vi "read_sample_results_files.vi"(8 "Error In":errorcluster, 10 "Sample":string, 11 "File Path":path) -> (0 "Error Out":errorcluster, 3 "Sample Results":T1)   [LabVIEW 2019]
uses:
  sample_results_cluster_typedef.ctl
  parameters_cluster_typedef.ctl
  writeable_section_parameters_cluster_typedef.ctl
  grain_results_cluster_typedef.ctl
panel:
  out "Exists?":bool
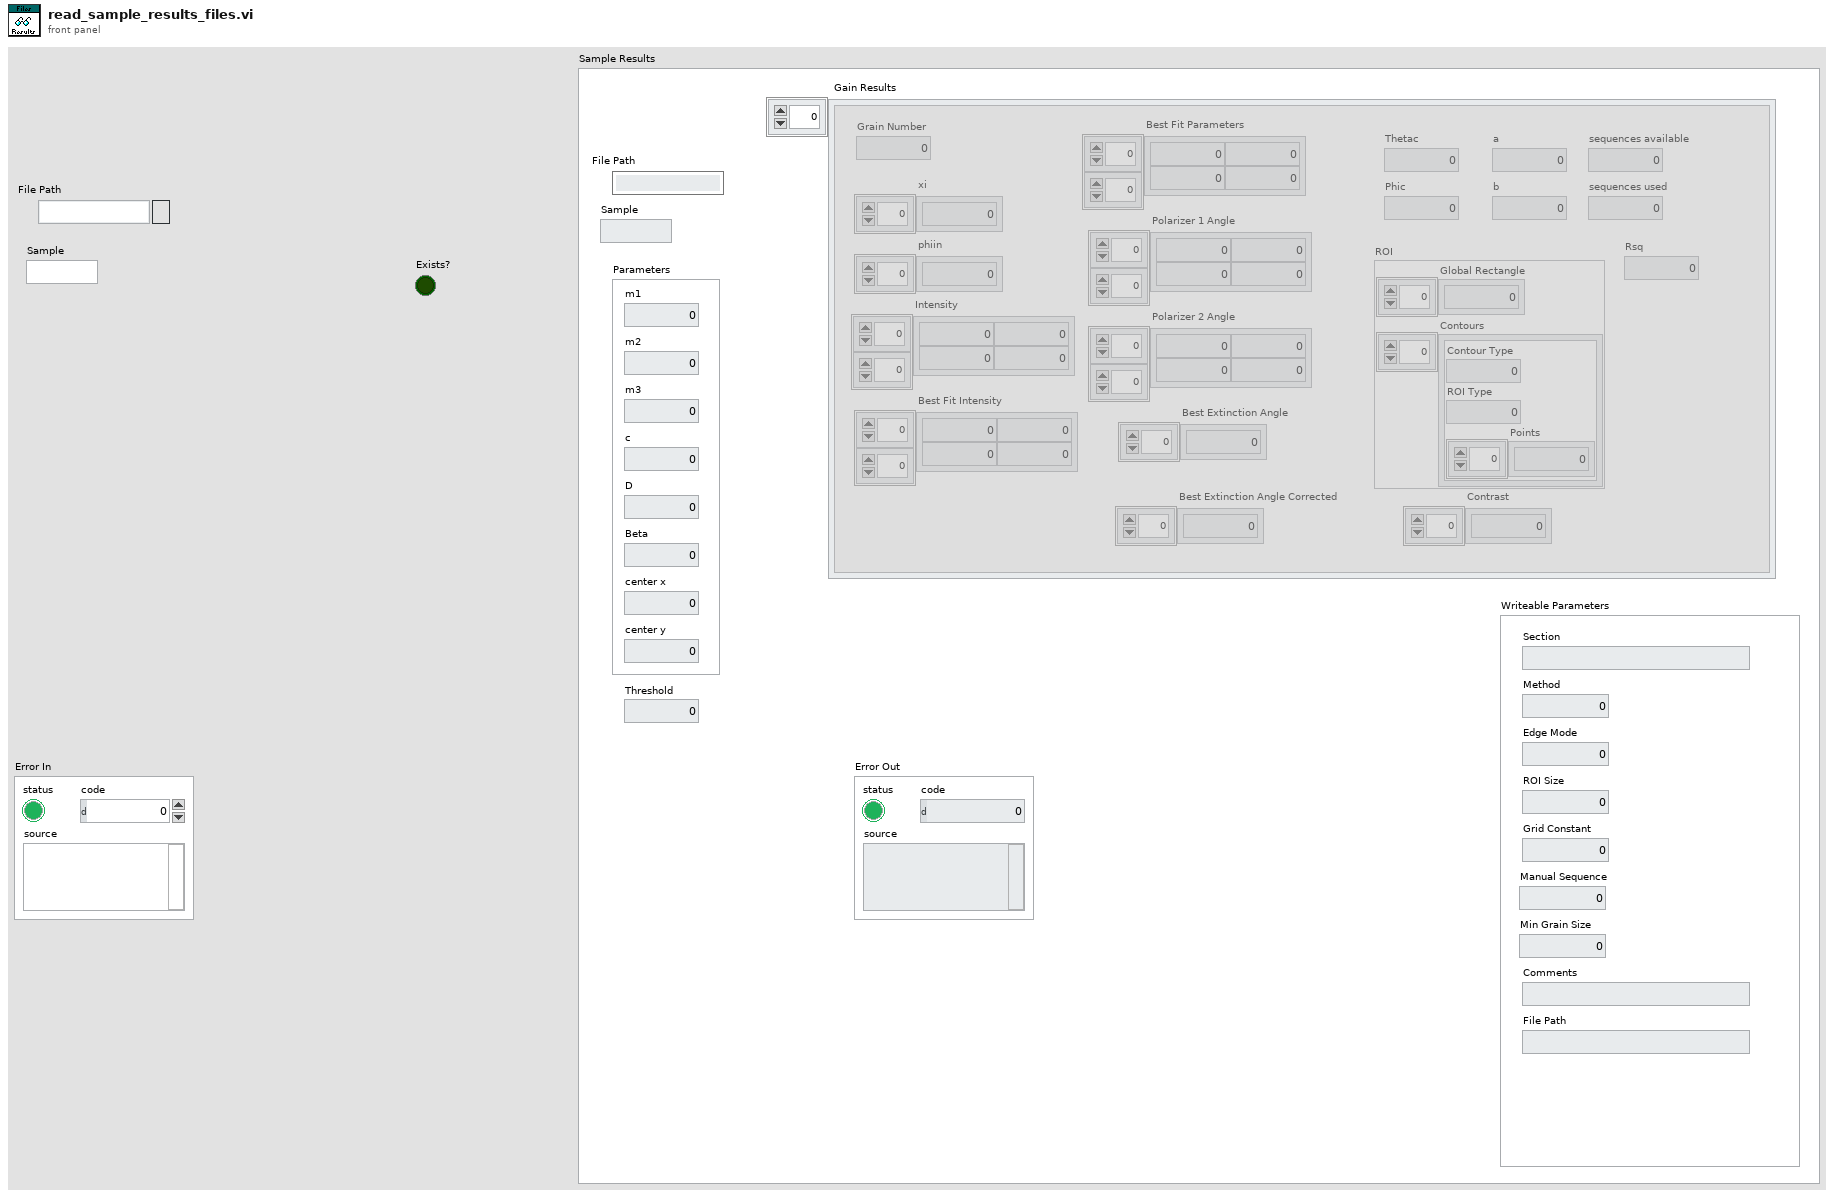
[diagram p1: front panel]
types:
  T1 = typedef "sample_results_cluster_typedef.ctl" = cluster{"File Path":string, "Sample":string, "Threshold":dbl, "Parameters":T2, "Writeable Parameters":T3, "Gain Results":T4[]}
  T2 = typedef "parameters_cluster_typedef.ctl" = cluster{"m1":dbl, "m2":dbl, "m3":dbl, "c":dbl, "D":dbl, "Beta":dbl, "center x":dbl, "center y":dbl}
  T3 = typedef "writeable_section_parameters_cluster_typedef.ctl" = cluster{"Section":string, "Method":i32, "Edge Mode":i32, "Grid Constant":i32, "Manual Sequence":i32, "ROI Size":i32, "Min Grain Size":dbl, "Comments":string, "File Path":string}
  T4 = typedef "grain_results_cluster_typedef.ctl" = cluster{"Grain Number":i32, "xi":dbl[], "phiin":dbl[], "Intensity":dbl[][], "Best Fit Intensity":dbl[][], "Best Fit Parameters":dbl[][], "Polarizer 1 Angle":dbl[][], "Polarizer 2 Angle":dbl[][], "Best Extinction Angle":dbl[], "Best Extinction Angle Corrected":dbl[], "Thetac":dbl, "Phic":dbl, "ROI":cluster{"Global Rectangle":i32[], "Contours":cluster{"Contour Type":u32, "ROI Type":u32, "Points":i32[]}[]}, "a":dbl, "b":dbl, "sequences available":dbl, "sequences used":dbl, "Contrast":dbl[], "Rsq":dbl}
  T5 = enum16{"open", "replace", "create", "open or create", "replace or create", "replace or create with confirmation"}
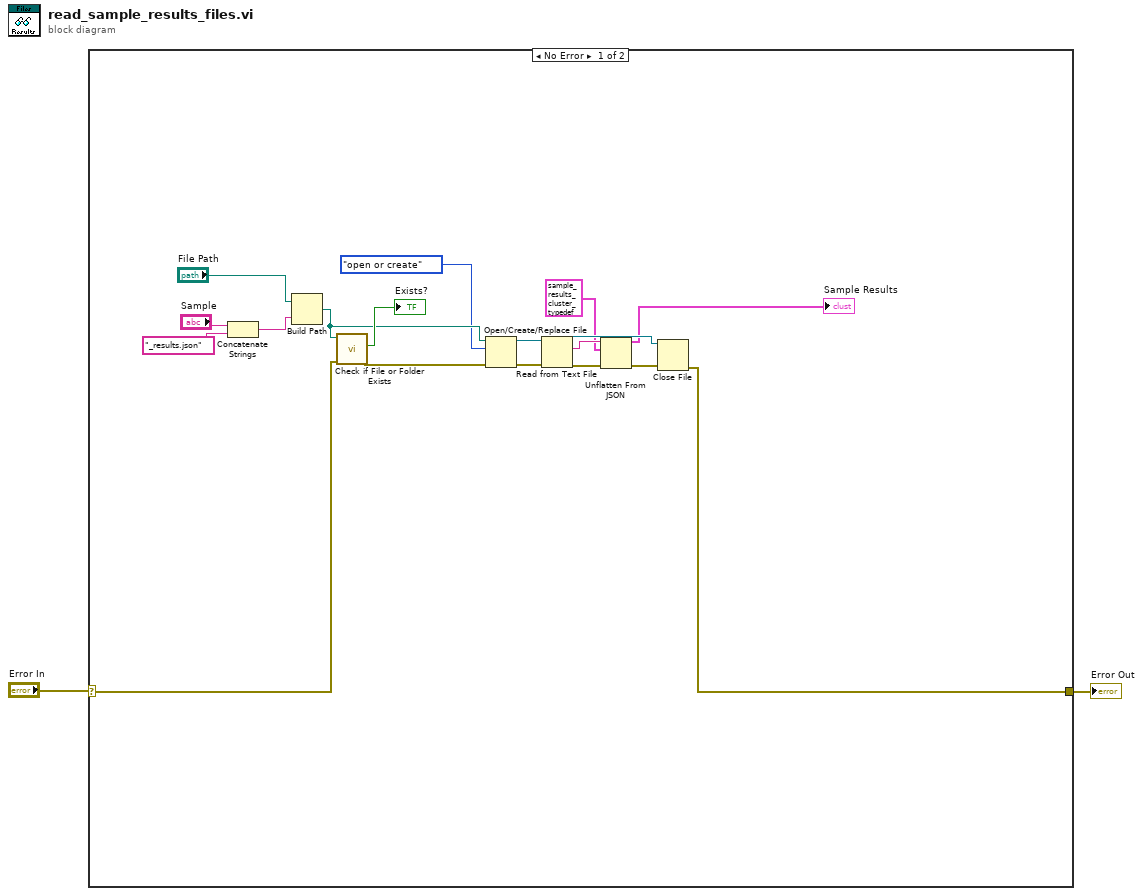
[diagram p0: block diagram]
diagram:
  n1 = case shown="No Error" "Error In" {
    selector: "Error In" -> [w15 w21]
    tunnel: [w3 w21] -> w1
    frame No Error {
      n2 = Concatenate Strings("Sample", "_results.json" ("string")) -> (w20:string)
      n3 = Build Path(base path="File Path", name or relative path=w20) -> (appended path=w7:path)
      n4 = call <vilib>:"Check if File or Folder Exists.vi"("error in (no error)"=w15, "path"=w7) -> ("error out"=w8:errorcluster, "file or folder exists?"=→"Exists?":bool)  [unwired: 7 in, 1 out]
      n5 = Open/Create/Replace File(file path (use dialog)=w7, error in=w8, operation (0:open)=T5."open or create") -> (refnum out=w13:refnum<file>, error out=w14:errorcluster)  [unwired: 3 in, 1 out]
      n6 = Read from Text File(file (use dialog)=w13, error in=w14) -> (refnum out=w9:refnum<file>, text=w12:string, error out=w11:errorcluster)  [unwired: 2 in, 1 out]
      n7 = Unflatten From JSON(JSON string=w12, type and defaults=T1 {"File Path"="", "Sample"="", "Threshold"=0.0, "Parameters"={"m1"=0.0, "m2"=0.0, "m3"=0.0, "c"=0.0, "D"=0.0, "Beta"=0.0, "center x"=0.0, "center y"=0.0}, "Writeable Parameters"={"Section"="", "Method"=0, "Edge Mode"=0, "Grid Constant"=0, "Manual Sequence"=0, "ROI Size"=0, "Min Grain Size"=0.0, "Comments"="", "File Path"=""}, "Gain Results"=[]} ("Sample Results"), error in (no error)=w11) -> (value=→"Sample Results":T1, error out=w10:errorcluster)  [unwired: 4 in]
      n8 = Close File(refnum=w9, error in=w10) -> (error out=w3:errorcluster)  [unwired: 1 out]
    }
    frame Error {
    }
  }
  "Error Out" <- w1
